vi "Fortschrittsbalken.vi"(0 "Slide ref":refnum<vi>, 2 "Gewichtung":dbl format="%#_13g", 5 "Gewichtung fortlaufend":dbl format="%#_13g", 9 "n":i32, 11 "i (0 bis n)":i32) -> (4 "Slide ref out":refnum<vi>, 6 "Gewichtung fortlaufend out":dbl)   [LabVIEW 2017, in "util.lvlib"]
uses:
  util.lvlib
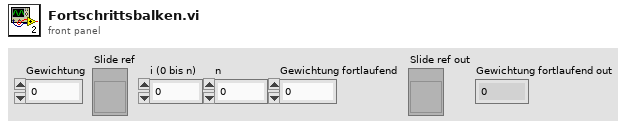
[diagram p1: front panel]
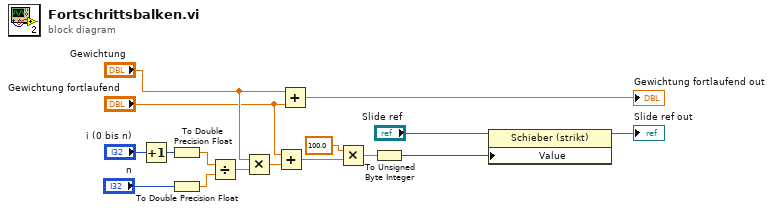
[diagram p0: block diagram]
diagram:
  n1 = Increment(x="i (0 bis n)") -> (x+1=w10:i32)
  n2 = To Double Precision Float(number=w10) -> (double precision float=w7:dbl)
  n3 = To Double Precision Float(number="n") -> (double precision float=w4:dbl)
  n4 = Divide(x=w7, y=w4) -> (x/y=w6:dbl)
  n5 = Multiply(x="Gewichtung", y=w6) -> (x*y=w2:dbl)
  n6 = Add(x="Gewichtung fortlaufend", y=w2) -> (x+y=w3:dbl)
  n7 = Add(x="Gewichtung", y="Gewichtung fortlaufend") -> (x+y=→"Gewichtung fortlaufend out":dbl)
  n8 = Multiply(x=100.0, y=w3) -> (x*y=w14:dbl)
  n9 = To Unsigned Byte Integer(number=w14) -> (unsigned 8bit integer=w15:u8)
  n10 = property on="Eigenschaftsknoten" class="Schieber (strikt)"(reference="Slide ref", "Value"=w15) -> (reference out=→"Slide ref out":refnum<vi>)  [unwired: 1 in, 1 out]
